vi "HAL camera start acquire.vi"(1 "error in":errorcluster) -> (0 "error out":errorcluster)   [LabVIEW 2016]
doc: "Starts an iXon acquisition (if not already running)"
uses:
  Atmcd32d.dll
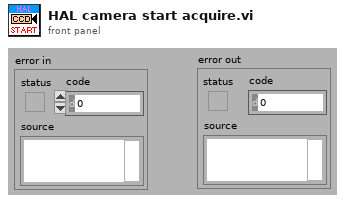
[diagram p1: front panel]
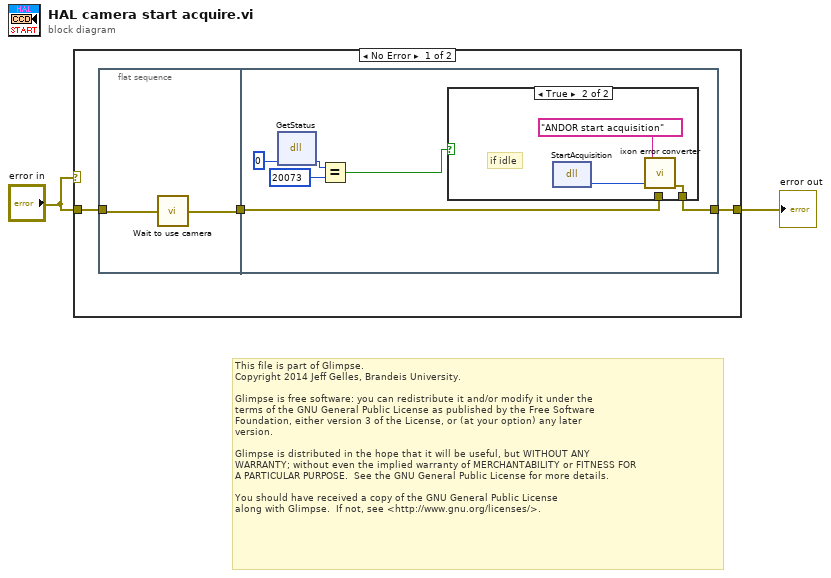
[diagram p0: block diagram]
diagram:
  # "This file is part of Glimpse. \nCopyright 2014 Jeff Gelles, Brandeis University.    \n\nGlimpse is free software: you can redistribute it and/or modify it under the \nterms of the GNU General Public License as published by the Free Software \nFoundation, either version 3 of the License, or (at your option) any later \nversion.\n\nGlimpse is distributed in the hope that it will be useful, but WITHOUT ANY \nWARRANTY; without even the implied warranty of MERCHANTABILITY or FITNESS FOR \nA PARTICULAR PURPOSE.  See the GNU General Public License for more details.\n\nYou should have received a copy of the GNU General Public License\nalong with Glimpse.  If not, see <http://www.gnu.org/licenses/>."
  n1 = case shown="No Error" "error in" {
    tunnel: "error in" -> [w5 w18]
    tunnel: [w4 w18] -> w2
    frame No Error {
      n2 = flat-sequence {
        tunnel: w5 -> [w6]
        tunnel: [w7] -> w3
        tunnel: [w8] -> w4
        tunnel: w3 -> [w13]
        frame #0 {
          n3 = call "Wait to use camera.vi"("error in"=w6) -> ("error out"=w7:errorcluster)
        }
        frame #1 {
          n4 = dll-call lib="ATMCD32D.DLL" fn="GetStatus" label="Call Library Function GetStatus"(u16 0) -> (w10:u32)  [unwired: 3 in, 3 out]
          n5 = Equal?(x=w10, y=u32 20073) -> (x = y?=w12:bool)
          n6 = case shown="True" w12 {
            tunnel: [w14 w15] -> w8
            tunnel: w13 -> [w14 _]
            frame False {
            }
            frame True {
              # "if idle"
              n7 = dll-call lib="ATMCD32D.DLL" fn="StartAcquisition" label="start acquisition"() -> ("return type"=w16:u32)  [unwired: 3 in, 2 out]
              n8 = call "ixon error converter.vi"("Andor error code"=w16, "source"="ANDOR start acquisition") -> ("error out"=w15:errorcluster)  [unwired: 5 out]
            }
          }
        }
      }
    }
    frame Error {
    }
  }
  "error out" <- w2
